vi "Initialize header map.vi"(8 "error in":errorcluster, 11 "header in":string) -> (0 "error out":errorcluster, 3 "header map":map{string, i32}(c390))   [LabVIEW 2020, in "Configuration_Helper.lvlib"]
uses:
  Configuration_Helper.lvlib
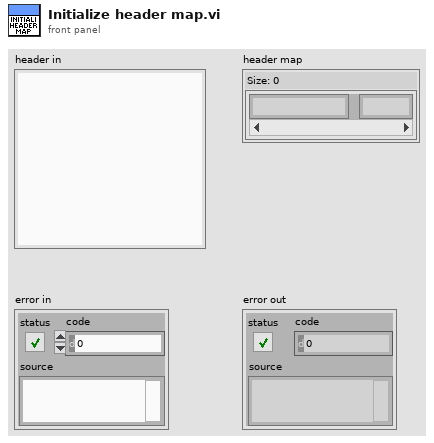
[diagram p1: front panel]
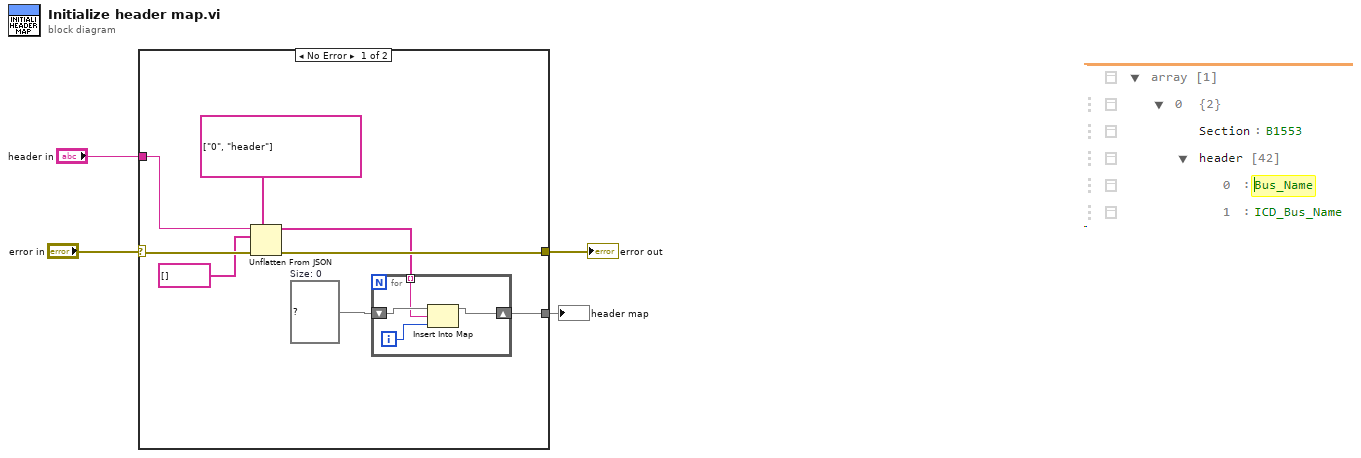
[diagram p0: block diagram]
diagram:
  n1 = case shown="No Error" "error in" {
    selector: "error in" -> [w11 w17]
    tunnel: [w8 w17] -> w3
    tunnel: "header in" -> [w12 _]
    tunnel: [w5 _] -> w1
    frame No Error {
      w7 = map{string, i32} {}  # Size: 0
      n2 = Unflatten From JSON(path=string[] ["0", "header"], JSON string=w12, type and defaults=string[] [] ("path"), error in (no error)=w11) -> (value=w6:string[], error out=w8:errorcluster)  [unwired: 3 in]
      n3 = for {
        shift-right: [w15] -> w5
        shift-left: w7 -> [w16]
        tunnel: w6 -> [w14] mode=indexing
        i -> [w13]
        n4 = Insert Into Map(map in=w16, key=w14, value=w13) -> (map out=w15:map{string, i32})  [unwired: 2 out]
      }
    }
    frame Error {
    }
  }
  "error out" <- w3
  "header map" <- w1
